vi "initHardware.vi"() -> (0 "error out":errorcluster, 1 "Encoders Task":refnum<k21>[](array[refnum]), 2 "Voltage Out":refnum<k21>, 5 "Tension Sensors":refnum<k21>)   [LabVIEW 2013]
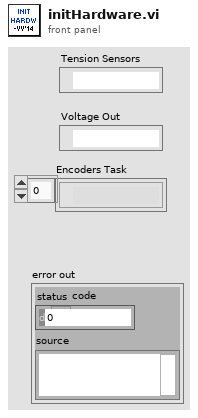
[diagram p1: front panel]
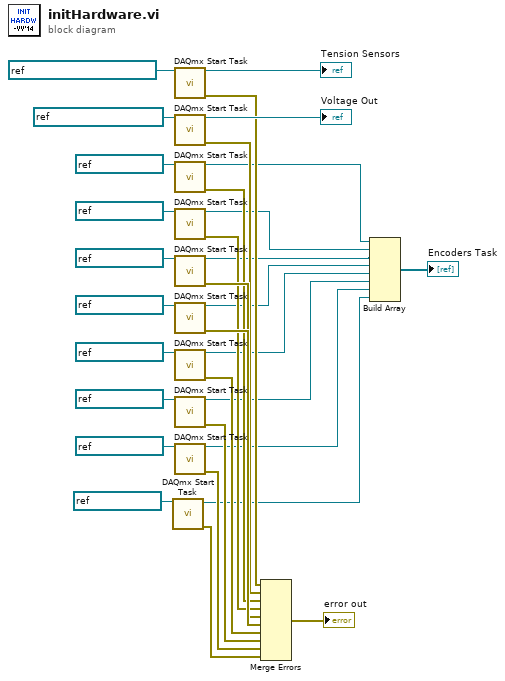
[diagram p0: block diagram]
diagram:
  n1 = call <vilib>:"DAQmx Start Task.vi"("task/channels in"=refnum<k21> "M8Encoder" ("DAQmx Task Name")) -> ("task out"=w1:refnum<k21>, "error out"=w2:errorcluster)  [unwired: 13 in]
  n2 = call <vilib>:"DAQmx Start Task.vi"("task/channels in"=refnum<k21> "TPAD_TenSen_PresSen" ("DAQmx Task Name")) -> ("task out"=→"Tension Sensors":refnum<k21>, "error out"=w21:errorcluster)  [unwired: 13 in]
  n3 = call <vilib>:"DAQmx Start Task.vi"("task/channels in"=refnum<k21> "tpadVoltageOutput" ("DAQmx Task Name")) -> ("task out"=→"Voltage Out":refnum<k21>, "error out"=w22:errorcluster)  [unwired: 13 in]
  n4 = call <vilib>:"DAQmx Start Task.vi"("task/channels in"=refnum<k21> "M1Encoder" ("DAQmx Task Name")) -> ("task out"=w11:refnum<k21>, "error out"=w23:errorcluster)  [unwired: 13 in]
  n5 = call <vilib>:"DAQmx Start Task.vi"("task/channels in"=refnum<k21> "M2Encoder" ("DAQmx Task Name")) -> ("task out"=w10:refnum<k21>, "error out"=w24:errorcluster)  [unwired: 13 in]
  n6 = call <vilib>:"DAQmx Start Task.vi"("task/channels in"=refnum<k21> "M3Encoder" ("DAQmx Task Name")) -> ("task out"=w9:refnum<k21>, "error out"=w25:errorcluster)  [unwired: 13 in]
  n7 = call <vilib>:"DAQmx Start Task.vi"("task/channels in"=refnum<k21> "M4Encoder" ("DAQmx Task Name")) -> ("task out"=w8:refnum<k21>, "error out"=w26:errorcluster)  [unwired: 13 in]
  n8 = call <vilib>:"DAQmx Start Task.vi"("task/channels in"=refnum<k21> "M5Encoder" ("DAQmx Task Name")) -> ("task out"=w7:refnum<k21>, "error out"=w27:errorcluster)  [unwired: 13 in]
  n9 = call <vilib>:"DAQmx Start Task.vi"("task/channels in"=refnum<k21> "M6Encoder" ("DAQmx Task Name")) -> ("task out"=w6:refnum<k21>, "error out"=w28:errorcluster)  [unwired: 13 in]
  n10 = call <vilib>:"DAQmx Start Task.vi"("task/channels in"=refnum<k21> "M7Encoder" ("DAQmx Task Name")) -> ("task out"=w5:refnum<k21>, "error out"=w29:errorcluster)  [unwired: 13 in]
  n11 = Merge Errors(w21, w22, w23, w24, w25, w26, w27, w28, w29, w2) -> (→"error out":errorcluster)
  n12 = Build Array(w11, w10, w9, w8, w7, w6, w5, w1) -> (→"Encoders Task":refnum<k21>[])
